vi "estruturas_controle.vi"() -> ()   [LabVIEW 2013]
panel:
  in  "stop":bool
  out "Off":bool
  out "On":bool
  in  "Ação":bool
  out "Array":dbl[](array[numeric])
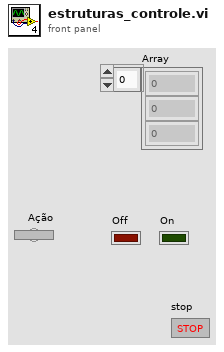
[diagram p1: front panel]
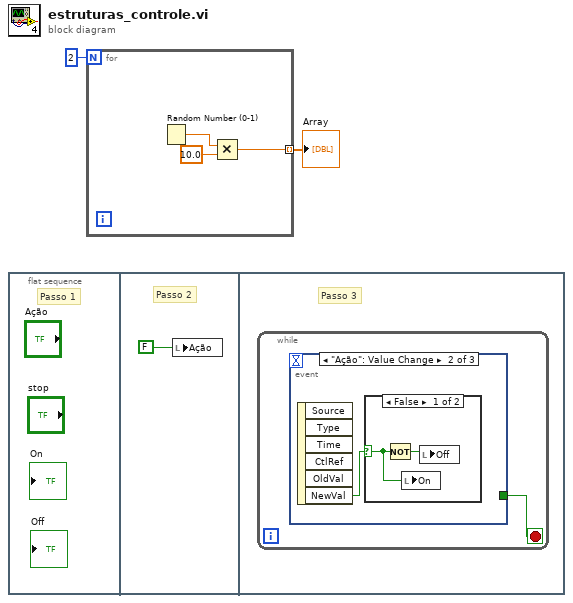
[diagram p0: block diagram]
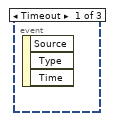
[diagram p2: hidden frame]
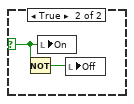
[diagram p3: hidden frame]
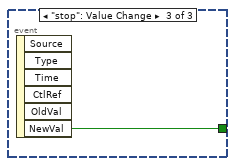
[diagram p4: hidden frame]
diagram:
  n1 = flat-sequence {
    frame #0 {
      # "Passo 1"
    }
    frame #1 {
      # "Passo 2"
      n2 = local write "Ação"(FALSE ("Boolean")) -> ()
    }
    frame #2 {
      # "Passo 3"
      n3 = while {
        stop <- w4 stop-if-true
        n4 = event shown="[1] \"Ação\": Value Change" {
          selector: _ -> [_ _ _]
          dyn-events: _ -> [_ _ _]
          timeout: _ -> [_ _ _]
          tunnel: [_ _ w10] -> w4
          event Timeout {
            n5 = event-data() -> ()  [unwired: 1 in, 3 out]
          }
          event "Ação": Value Change {
            n6 = event-data() -> ("NewVal"=w5:bool)  [unwired: 1 in, 5 out]
            n7 = case shown="False" w5 {
              selector: w5 -> [w6 w9]
              frame False {
                n8 = Not(x=w6) -> (.not. x?=w7:bool)
                n9 = local write "On"(w6) -> ()
                n10 = local write "Off"(w7) -> ()
              }
              frame True {
                n11 = Not(x=w9) -> (.not. x?=w8:bool)
                n12 = local write "On"(w9) -> ()
                n13 = local write "Off"(w8) -> ()
              }
            }
          }
          event "stop": Value Change {
            n14 = event-data() -> ("NewVal"=w10:bool)  [unwired: 1 in, 5 out]
          }
        }
      }
    }
  }
  n15 = for {
    N: 2 -> [_]
    tunnel: [w11] -> w1 mode=indexing
    n16 = Random Number (0-1)() -> (number: 0 to 1=w12:dbl)
    n17 = Multiply(x=w12, y=10.0) -> (x*y=w11:dbl)
  }
  "Array" <- w1
